vi "WFDC Get XY Drift.vi"(0 "Ref Images":T1[](array[typedef]), 2 "Half Shift":i32=7, 5 "Current Image":u16[][](array[numeric]), 7 "CC Threshold":dbl, 9 "Roundness Ratio":dbl, 11 "Error In":errorcluster) -> (4 "Axis 1 Drift (px)":dbl, 6 "Axis 2 Drift (px)":dbl, 8 "CC Image":dbl[][](array[numeric]), 10 "CC Fit":dbl[][](array[numeric]), 15 "Error Out":errorcluster)   [LabVIEW 2020]
uses:
  <vilib>/vision/Image Controls.llb/IMAQ Image.ctl
  WFDC DLL and Testing/Visual Studio NCC Max Shift DLL/x64/Release/VSmaxShiftNCC.dll
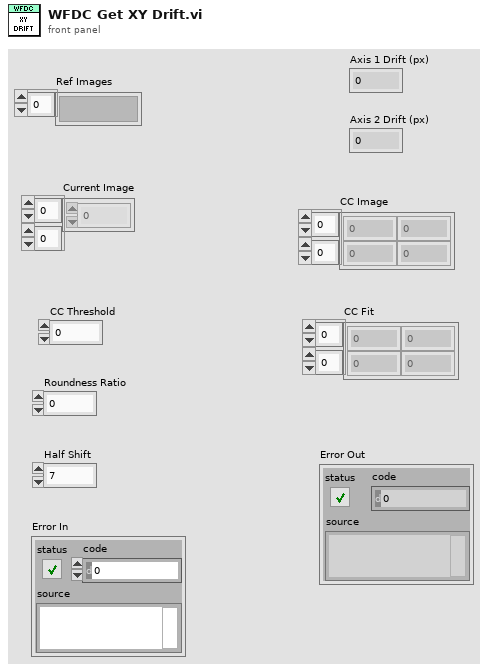
[diagram p1: front panel]
types:
  T1 = typedef "IMAQ Image.ctl" = refnum<image>
  T2 = typedef "2D Gaussian - Best Fit Parameters.ctl" = cluster{"Amplitude":dbl, "X Position":dbl, "Y Position":dbl, "X Width":dbl, "Y Width":dbl, "Offset":dbl}
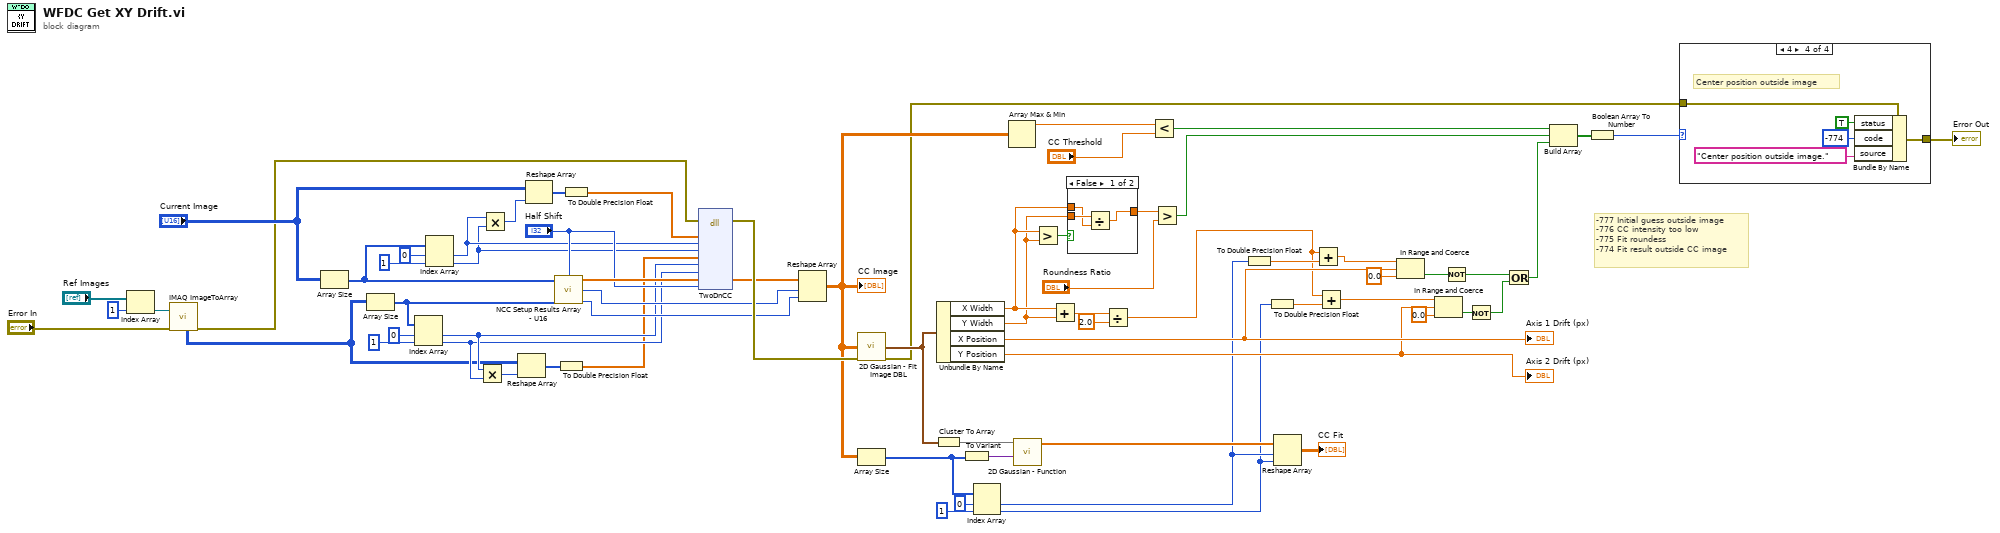
[diagram p0: block diagram]
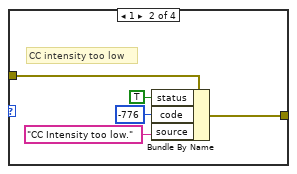
[diagram p3: hidden frame]
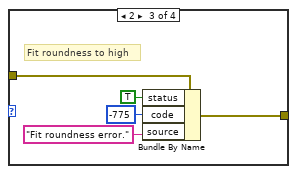
[diagram p4: hidden frame]
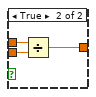
[diagram p5: hidden frame]
diagram:
  # "-777 Initial guess outside image\n-776 CC intensity too low\n-775 Fit roundess\n-774 Fit result outside CC image"
  n1 = Index Array(array="Ref Images", index=1) -> (element=w42:T1)
  n2 = call "IMAQ ImageToArray"("error in (no error)"="Error In", "Image"=w42) -> ("Image Pixels (U16)"=w41:u16[][], "error out"=w67:errorcluster)  [unwired: 2 in, 3 out]
  n3 = Array Size(array="Current Image") -> (size(s)=w50:i32[])
  n4 = Array Size(array=w41) -> (size(s)=w60:i32[])
  n5 = Index Array(array=w60, index #1=0 ("index"), index #2=1 ("index")) -> (element #1=w57:i32, element #2=w56:i32)
  n6 = Index Array(array=w50, index #1=0 ("index"), index #2=1 ("index")) -> (element #1=w47:i32, element #2=w46:i32)
  n7 = Multiply(x=w57, y=w56) -> (x*y=w55:i32)
  n8 = Multiply(x=w47, y=w46) -> (x*y=w45:i32)
  n9 = Reshape Array(w41, w55) -> (w54:u16[])
  n10 = Reshape Array("Current Image", w45) -> (w49:u16[])
  n11 = call "NCC Setup Results Array - U16.vi"("Image 01 Size"=w50, "Half Shift"="Half Shift", "Image 02 Size"=w60) -> ("NCC Results Array"=w65:dbl[], "Result Rows"=w62:i32, "Result Columns"=w63:i32)  [unwired: 10 in]
  n12 = To Double Precision Float(number=w54) -> (double precision float=w53:dbl[])
  n13 = To Double Precision Float(number=w49) -> (double precision float=w48:dbl[])
  n14 = dll-call lib="C:/Users/George Sirinakis/Documents/Microscope-Control/Microscope Modules/Wide Field Drift Correction/WFDC DLL and Testing/Visual Studio NCC Max Shift DLL/x64/Release/VSmaxShiftNCC.dll" fn="TwoDnCC"(error in=w67, "im01"=w48, "im01rowSize"=w47, "im01colSize"=w46, "im02"=w53, "im02rowSize"=w57, "im02ColSize"=w56, "theResult"=w65, "halfShift"="Half Shift") -> (error out=w66:errorcluster, "theResult"=w64:dbl[])  [unwired: 10 in, 1 out]
  n15 = Reshape Array(w64, w62, w63) -> (w32:dbl[][])
  "CC Image" <- w32
  n16 = call "2D Gaussian - Fit Image DBL.vi"("Image In (DBL)"=w32, "Error In"=w66) -> ("Best Fit Params"=w40:T2, "Error Out"=w14:errorcluster)  [unwired: 12 in]
  n17 = Array Size(array=w32) -> (size(s)=w37:i32[])
  n18 = Cluster To Array(cluster=w40) -> (array=w35:dbl[])
  n19 = Unbundle By Name(w40) -> ("X Width"=w7:dbl, "Y Width"=w6:dbl, "X Position"=w29:dbl, "Y Position"=w28:dbl)
  "Axis 2 Drift (px)" <- w28
  "Axis 1 Drift (px)" <- w29
  n20 = To Variant(anything=w37) -> (Variant=w34:variant)
  n21 = Index Array(array=w37, index #1=0 ("index"), index #2=1 ("index")) -> (element #1=w12:i32, element #2=w11:i32)
  n22 = Array Max & Min(array=w32) -> (max value=w31:dbl)  [unwired: 3 out]
  n23 = call "2D Gaussian - Function.vi"("data"=w34, "a"=w35) -> ("f(X,a)"=w36:dbl[])  [unwired: 2 in, 2 out]
  n24 = Greater?(x=w7, y=w6) -> (0:w23:bool)
  n25 = Add(x=w7, y=w6) -> (x+y=w5:dbl)
  n26 = case shown="False" w23 {
    tunnel: w7 -> [w71 w75]
    tunnel: w6 -> [w72 w74]
    tunnel: [w70 w73] -> w22
    frame False {
      n27 = Divide(x=w72, y=w71) -> (x/y=w70:dbl)
    }
    frame True {
      n28 = Divide(x=w75, y=w74) -> (x/y=w73:dbl)
    }
  }
  n29 = Divide(x=w5, y=2.0) -> (x/y=w3:dbl)
  n30 = Less?(x=w31, y="CC Threshold") -> (x < y?=w19:bool)
  n31 = Greater?(x=w22, y="Roundness Ratio") -> (0:w18:bool)
  n32 = To Double Precision Float(number=w12) -> (double precision float=w10:dbl)
  n33 = To Double Precision Float(number=w11) -> (double precision float=w9:dbl)
  n34 = Reshape Array(w36, w12, w11) -> (→"CC Fit":dbl[][])
  n35 = Add(x=w3, y=w10) -> (x+y=w2:dbl)
  n36 = Add(x=w3, y=w9) -> (x+y=w1:dbl)
  n37 = In Range and Coerce(upper limit=w2, x=w29, lower limit=0.0) -> (In Range?=w25:bool)  [unwired: 1 out]
  n38 = In Range and Coerce(upper limit=w1, x=w28, lower limit=0.0) -> (In Range?=w24:bool)  [unwired: 1 out]
  n39 = Not(x=w25) -> (.not. x?=w21:bool)
  n40 = Not(x=w24) -> (.not. x?=w20:bool)
  n41 = Or(x=w21, y=w20) -> (x .or. y?=w17:bool)
  n42 = Build Array(w19, w18, w17) -> (w16:bool[])
  n43 = Boolean Array To Number(Boolean array=w16) -> (number=w15:u32)
  n44 = case shown="4" w15 {
    tunnel: w14 -> [w76 w81 w83 w88]
    tunnel: [w76 w77 w82 w87] -> w13
    frame Default {
    }
    frame 1 {
      # "CC intensity too low"
      n45 = Bundle By Name(cluster=w81, "status"=TRUE, "code"=-776, "source"="CC Intensity too low.") -> (w77:errorcluster)
    }
    frame 2 {
      # "Fit roundness to high"
      n46 = Bundle By Name(cluster=w83, "status"=TRUE, "code"=-775, "source"="Fit roundness error.") -> (w82:errorcluster)
    }
    frame 4 {
      # "Center position outside image"
      n47 = Bundle By Name(cluster=w88, "status"=TRUE, "code"=-774, "source"="Center position outside image.") -> (w87:errorcluster)
    }
  }
  "Error Out" <- w13
